vi "VL Type.vi"(8 "error in (no error)":errorcluster, 11 "Task in":refnum<class "Task.lvclass">) -> (0 "error out":errorcluster, 2 "VL Type":T1, 3 "Task out":refnum<class "Task.lvclass">)   [LabVIEW 2020, in "VolatusConfig.lvlib" / "Task.lvclass"]
uses:
  Task.lvclass
  Meta Type.ctl
  VolatusConfig.lvlib
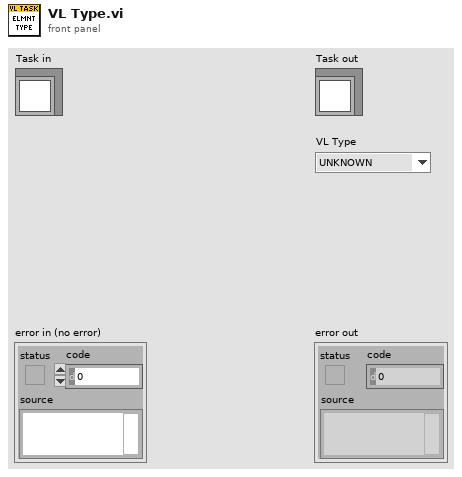
[diagram p1: front panel]
types:
  T1 = typedef "VolatusConfig.lvlib/Meta Type.ctl" = enum16{"UNKNOWN", "VL_System", "VL_Cluster", "VL_Node", "VL_Task", "VL_Group", "VL_Channel", "VL_Task_List", "VL_Scaling", "VL_Sensor", "VL_Sensor_List", "VL_Scale"}
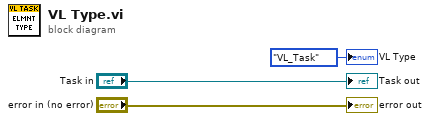
[diagram p0: block diagram]
diagram:
  "error out" <- "error in (no error)"
  "Task out" <- "Task in"
  "VL Type" <- Meta_Type."VL_Task" ("VL Type")
